vi "Config-Termination.vi"(8 "error in (no error)":errorcluster, 10 "Def-PreConfig-Termination":T1, 11 "CAN-NI in":refnum<class "CAN-NI.lvclass">) -> (0 "error out":errorcluster, 3 "CAN-NI out":refnum<class "CAN-NI.lvclass">)   [LabVIEW 2019, in "CAN-NI.lvlib" / "CAN-NI.lvclass"]
uses:
  CAN-NI.lvclass
  CAN-Interface/TypeDef/Def-PreConfig-Termination.ctl
  CAN-Interface/TypeDef/Def-Termination.ctl
  <resource>/objmgr/xnet.rc
  CAN-Interface/Class-Interface.lvclass
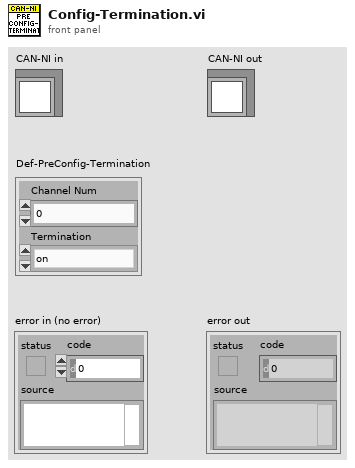
[diagram p1: front panel]
types:
  T1 = typedef "CAN-Interface.lvlib/Class-Interface.lvclass/Def-PreConfig-Termination.ctl" = cluster{"Channel Num":u32, "Termination":T2}
  T2 = typedef "CAN-Interface.lvlib/Class-Interface.lvclass/Def-Termination.ctl" = enum8{"on", "off"}
  T3 = typedef "CAN-NI.lvlib/CAN-NI.lvclass/ChannelProperty.ctl" = cluster{"CAN-cluster":refnum<k21>, "CAN-Frames":refnum<k21>[], "Termination":T2, "Transmit Mode":T4, "Frame Out Session":refnum<k21>, "Frame In Session":refnum<k21>, "Protocol":T5}
  T4 = typedef "CAN-Interface.lvlib/Class-Interface.lvclass/Def-Transmit Mode.ctl" = enum16{"Queued", "Stream"}
  T5 = typedef "CAN-Interface.lvlib/Class-Interface.lvclass/Def-Protocol.ctl" = enum16{"CAN", "CAN FD"}
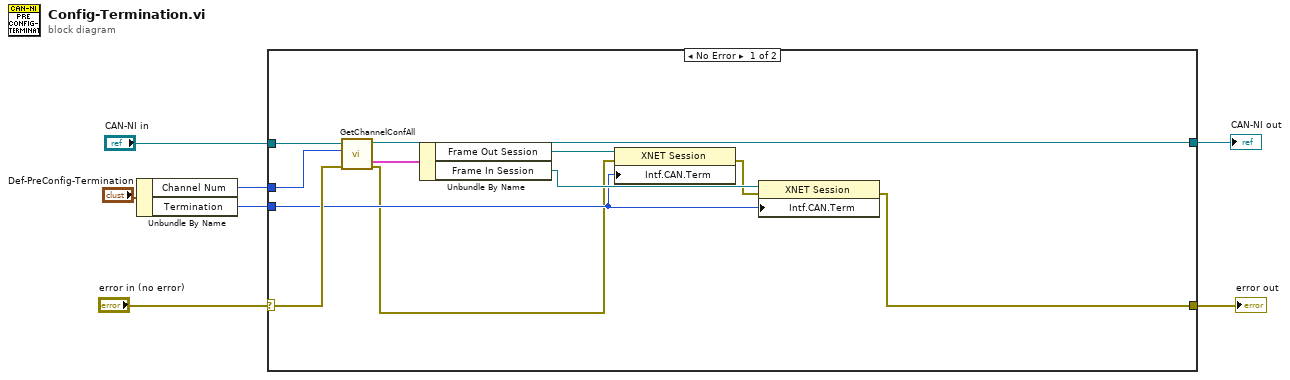
[diagram p0: block diagram]
diagram:
  n1 = Unbundle By Name("Def-PreConfig-Termination") -> ("Channel Num"=w2:u32, "Termination"=w1:T2)
  n2 = case shown="No Error" "error in (no error)" {
    selector: "error in (no error)" -> [w16 w19]
    tunnel: "CAN-NI in" -> [w18 w20]
    tunnel: [w14 w20] -> w5
    tunnel: [w8 w19] -> w4
    tunnel: w2 -> [w17 _]
    tunnel: w1 -> [w11 _]
    frame No Error {
      n3 = call "GetChannelConfAll.vi"("error in"=w16, "Channel Num"=w17, "CAN-NI"=w18) -> ("error out"=w10:errorcluster, "ChannelProperty"=w15:T3, "CAN-NI"=w14:refnum<class "CAN-NI.lvclass">)  [unwired: 6 in]
      n4 = Unbundle By Name(w15) -> ("Frame Out Session"=w13:refnum<k21>, "Frame In Session"=w12:refnum<k21>)
      n5 = property class="XNET Session"(reference=w13, error in=w10, "Intf.CAN.Term"=w11) -> (error out=w9:errorcluster)  [unwired: 1 out]
      n6 = property class="XNET Session"(reference=w12, error in=w9, "Intf.CAN.Term"=w11) -> (error out=w8:errorcluster)  [unwired: 1 out]
    }
    frame Error {
    }
  }
  "error out" <- w4
  "CAN-NI out" <- w5
